vi "Variable Launch Angle Trajectory.vi"() -> ()   [LabVIEW 2016]
panel:
  out "Launch Angle 2":dbl
  out "Trajectory Graph":cluster{"Y Values":dbl[], "Y Values":dbl[]}[](graph)
  out "Launch Angle 1":dbl
  in  "Vertical Distance":dbl(slide) scale=0.0..10.0
  in  "Horizontal Distance":dbl(slide) scale=0.0..10.0
  in  "Launch Velocity":dbl(slide) scale=0.0..10.0
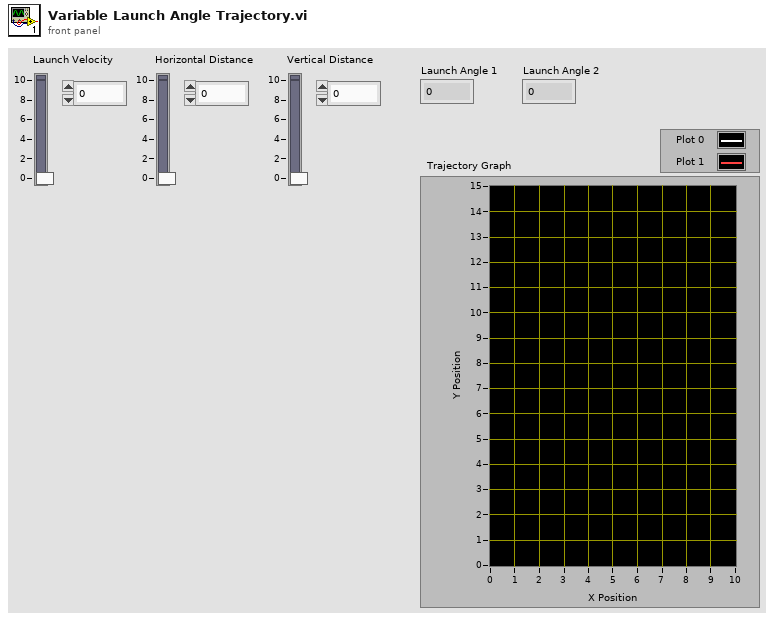
[diagram p1: front panel]
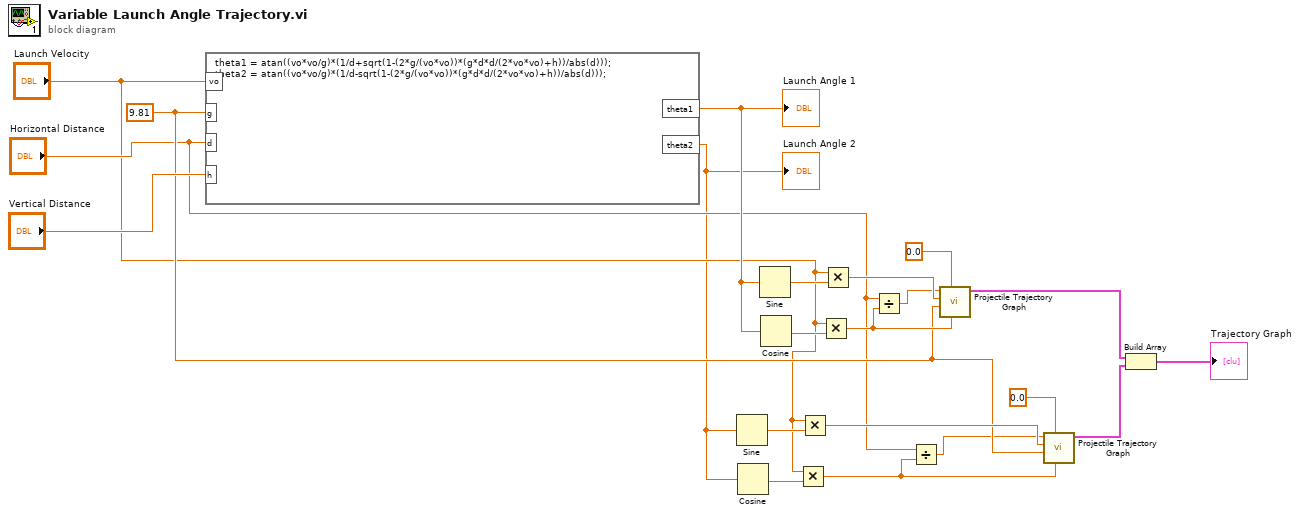
[diagram p0: block diagram]
diagram:
  w9 = 9.81 ("input variable")
  n1 = formula code="theta1 = atan((vo*vo/g)*(1/d+sqrt(1-(2*g/(vo*vo))*(g*d*d/(2*vo*vo)+h))/abs(d)));\ntheta2 = atan((vo*vo/g)*(1/d-sqrt(1-(2*g/(vo*vo))*(g*d*d/(2*vo*vo)+h))/abs(d)));"("vo"="Launch Velocity", "g"=w9, "d"="Horizontal Distance", "h"="Vertical Distance") -> ("theta1"=w11:dbl, "theta2"=w1:dbl)
  "Launch Angle 1" <- w11
  "Launch Angle 2" <- w1
  n2 = Sine(x=w1) -> (sin(x)=w15:dbl)
  n3 = Cosine(x=w1) -> (cos(x)=w14:dbl)
  n4 = Sine(x=w11) -> (sin(x)=w21:dbl)
  n5 = Cosine(x=w11) -> (cos(x)=w20:dbl)
  n6 = Multiply(x="Launch Velocity", y=w14) -> (x*y=w5:dbl)
  n7 = Multiply(x="Launch Velocity", y=w15) -> (x*y=w13:dbl)
  n8 = Multiply(x="Launch Velocity", y=w20) -> (x*y=w17:dbl)
  n9 = Multiply(x="Launch Velocity", y=w21) -> (x*y=w19:dbl)
  n10 = Divide(x="Horizontal Distance", y=w17) -> (x/y=w10:dbl)
  n11 = Divide(x="Horizontal Distance", y=w5) -> (x/y=w3:dbl)
  n12 = call "Projectile Trajectory Graph.vi"("X Velocity"=w17, "Initial Height"=0.0, "Gravitational Acceleration"=w9, "Initial Y Velocity"=w19, "End Time"=w10) -> ("Trajectory Graph"=w8:cluster{"Y Values":dbl[], "Y Values":dbl[]})  [unwired: 6 in]
  n13 = call "Projectile Trajectory Graph.vi"("X Velocity"=w5, "Initial Height"=0.0, "Gravitational Acceleration"=w9, "Initial Y Velocity"=w13, "End Time"=w3) -> ("Trajectory Graph"=w7:cluster{"Y Values":dbl[], "Y Values":dbl[]})  [unwired: 6 in]
  n14 = Build Array(w8, w7) -> (→"Trajectory Graph":cluster{"Y Values":dbl[], "Y Values":dbl[]}[])
